vi "Periodic Message Filter in CSM Tool.vi"(5 "Remove Immediately?(F)":bool, 7 "reset?":bool, 8 "Settings":T4={"threashold(#/s)"=2.0, "Check Peroid(s)"=1.0}, 11 "Cross CSM Data":T1={"Name(\"\" to use uuid)"="CSM Tiny", "Current State"="UI: Refresh Buttons", "Arguments"="", "Source Message"={"‘State"="", "’Arguments"="", "’Error"={"status"=FALSE, "code"=0, "source"=""}}, "Source Module"="<end>", "Complete(T)/Start(F)"=TRUE, "LogType"=enum."State Change"}) -> (0 "Filtered":bool, 1 "additional Info":string[](array[string]), 3 "Cross CSM Data out":T1={"Name(\"\" to use uuid)"="", "Current State"="", "Arguments"="", "Source Message"={"‘State"="", "’Arguments"="", "’Error"={"status"=FALSE, "code"=0, "source"=""}}, "Source Module"="", "Complete(T)/Start(F)"=FALSE, "LogType"=enum."State Change"}, 4 "Filtered Status":string[](array[string]))   [LabVIEW 2017, in "csm-tool-support.lvlib"]
uses:
  csm-tool-support.lvlib
  _Support/Typedef/_CSM_GlobalLog_MSG.ctl
  _Support/Typedef/_CSM_Response Source Message.ctl
  _Support/Typedef/_CSM_GlobalLog_MSG_TYPE.ctl
  Communicable State Machine.lvlib
  _Support/GlobalEvent/LogFilter/LogFilter.lvclass
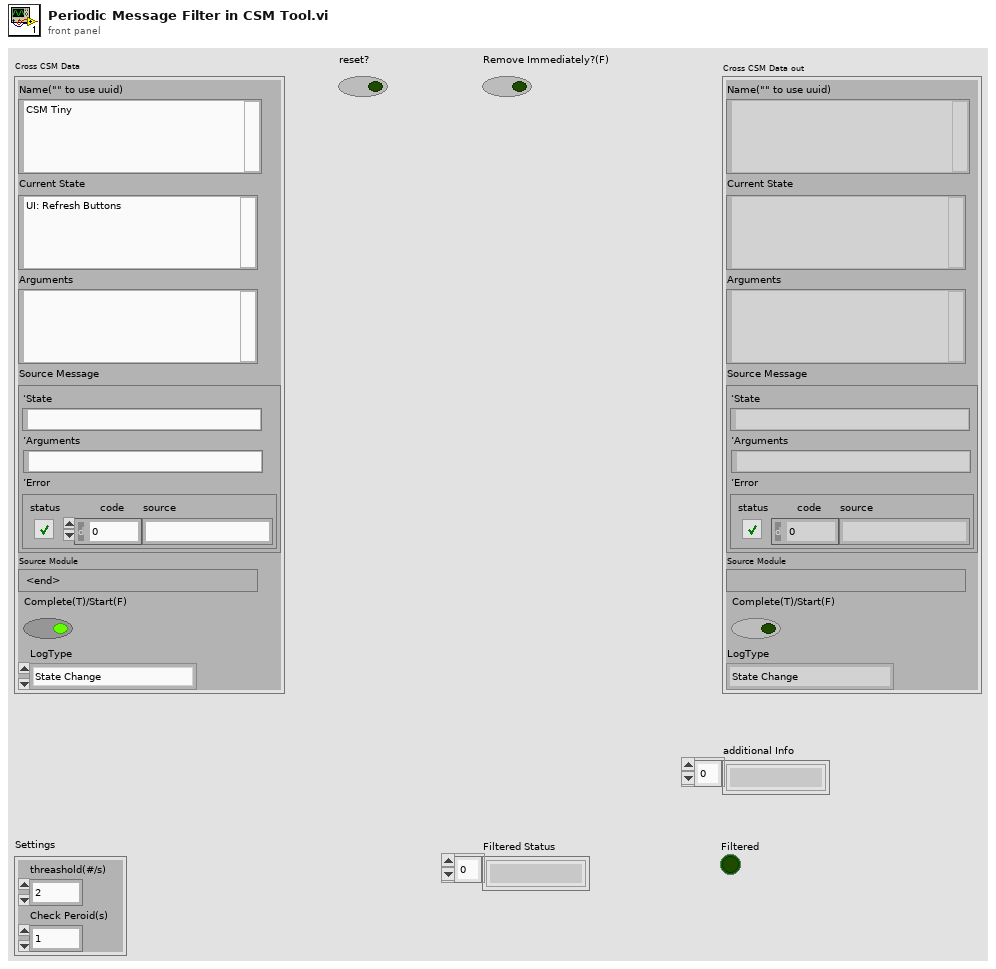
[diagram p1: front panel]
types:
  T1 = typedef "Communicable State Machine.lvlib/_CSM_GlobalLog_MSG.ctl" = cluster{"Name(\"\" to use uuid)":string, "Current State":string, "Arguments":string, "Source Message":T2, "Source Module":string, "Complete(T)/Start(F)":bool, "LogType":T3}
  T2 = typedef "Communicable State Machine.lvlib/_CSM_Response Source Message.ctl" = cluster{"‘State":string, "’Arguments":string, "’Error":errorcluster}
  T3 = typedef "Communicable State Machine.lvlib/_CSM_GlobalLog_MSG_TYPE.ctl" = enum16{"User Log", "State Change", "Status", "Interrupt", "Register", "Unregister", "Error Log", "Module Created", "Module Destroyed"}
  T4 = cluster{"threashold(#/s)":dbl, "Check Peroid(s)":dbl}
  T5 = cluster{"String":string, "Count":i64, "since":timestamp}[]
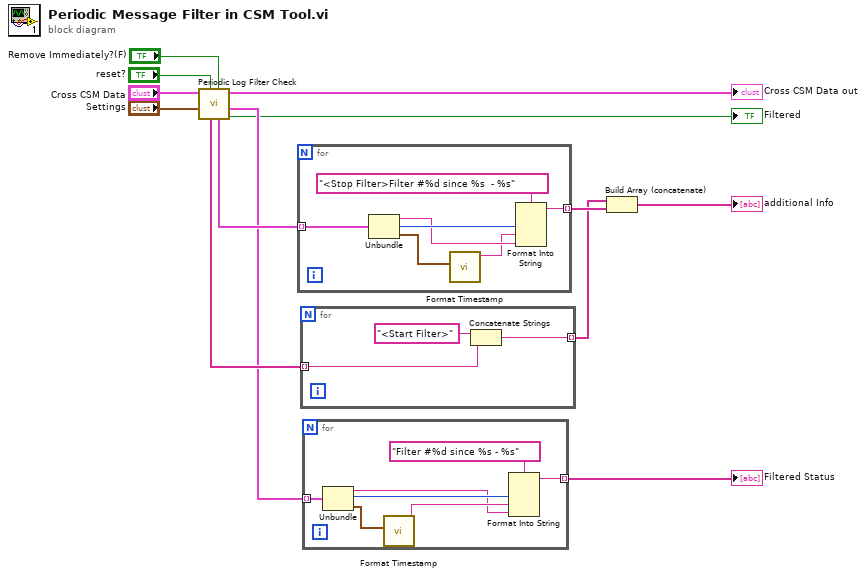
[diagram p0: block diagram]
diagram:
  n1 = call "Periodic Log Filter Check.vi"("Remove Immediately?(F)"="Remove Immediately?(F)", "reset?"="reset?", "Settings"="Settings", "Cross CSM Data"="Cross CSM Data") -> ("Filtered"=→"Filtered":bool, "Filtered Status"=w5:T5, "Cross CSM Data out"=→"Cross CSM Data out":T1, "removed info"=w12:T5, "added Info"=w13:string[])  [unwired: 3 in]
  n2 = for {
    tunnel: w12 -> [w15] mode=indexing
    tunnel: [w14] -> w11 mode=indexing
    n3 = Unbundle(w15) -> ("String"=w18:string, "Count"=w19:i64, "since"=w17:timestamp)
    n4 = call "Format Timestamp.vi"("timestamp"=w17) -> ("String"=w16:string)  [unwired: 10 in]
    n5 = Format Into String(format string="<Stop Filter>Filter #%d since %s  - %s", w19, w16, w18) -> (resulting string=w14:string)  [unwired: 2 in, 1 out]
  }
  n6 = for {
    tunnel: w13 -> [w22] mode=indexing
    tunnel: [w21] -> w10 mode=indexing
    n7 = Concatenate Strings("<Start Filter>" ("Current State"), w22) -> (w21:string)
  }
  n8 = for {
    tunnel: w5 -> [w29] mode=indexing
    tunnel: [w30] -> w4 mode=indexing
    n9 = Unbundle(w29) -> ("String"=w24:string, "Count"=w28:i64, "since"=w26:timestamp)
    n10 = call "Format Timestamp.vi"("timestamp"=w26) -> ("String"=w25:string)  [unwired: 10 in]
    n11 = Format Into String(format string="Filter #%d since %s - %s", w28, w25, w24) -> (resulting string=w30:string)  [unwired: 2 in, 1 out]
  }
  "Filtered Status" <- w4
  n12 = Build Array (concatenate)(w10, w11) -> (→"additional Info":string[])
